vi "SPI_GetThreeWire.vi"(5 "Device":i32, 7 "Bus":i32=1, 8 "error in":errorcluster) -> (0 "error out":errorcluster, 6 "Three Wire":bool)   [LabVIEW 2014, in "GPIO.lvlib"]
doc: "Reads whether or not the SI/SO lines for the specified SPI device are shared."
uses:
  GPIO.lvlib
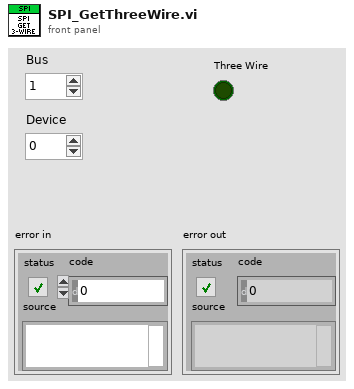
[diagram p1: front panel]
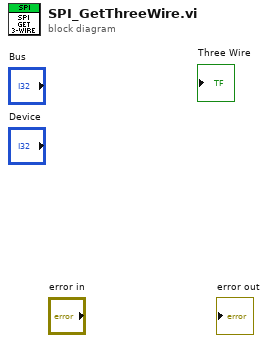
[diagram p0: block diagram]
diagram:
